vi "DC_Measurement.vi"(8 "stop":bool, 10 "millisecond multiple":u32, 11 "task/channels in":refnum<k21>="PTS_CAB1k_DCV") -> (0 "XY Graph":cluster{dbl[], dbl[]}(graph))   [LabVIEW 2021]
uses:
  <vilib>/DAQmx/read.llb/DAQmx Read (Analog 1D Wfm NChan NSamp).vi
  <vilib>/DAQmx/miscellaneous.llb/DAQmx Fill In Error Info.vi
  <vilib>/measure/madcrms.llb/Averaged DC-RMS for N Chan.vi
  <vilib>/measure/madcrms.llb/Basic Averaged DC-RMS for N Chan.vi
  <vilib>/measure/NI_MAPro.lvlib
panel:
  out "Waveform Graph":dbl[](graph)
  out "Array":dbl[](array[numeric])
  out "cycle average":dbl[](array[numeric]) format="%.2p"
  out "Raw Readings":waveform(dbl)[](graph)
  out "DC value waveforms":waveform(dbl)[](array[waveform])
  out "RMS value waveforms":waveform(dbl)[](array[waveform])
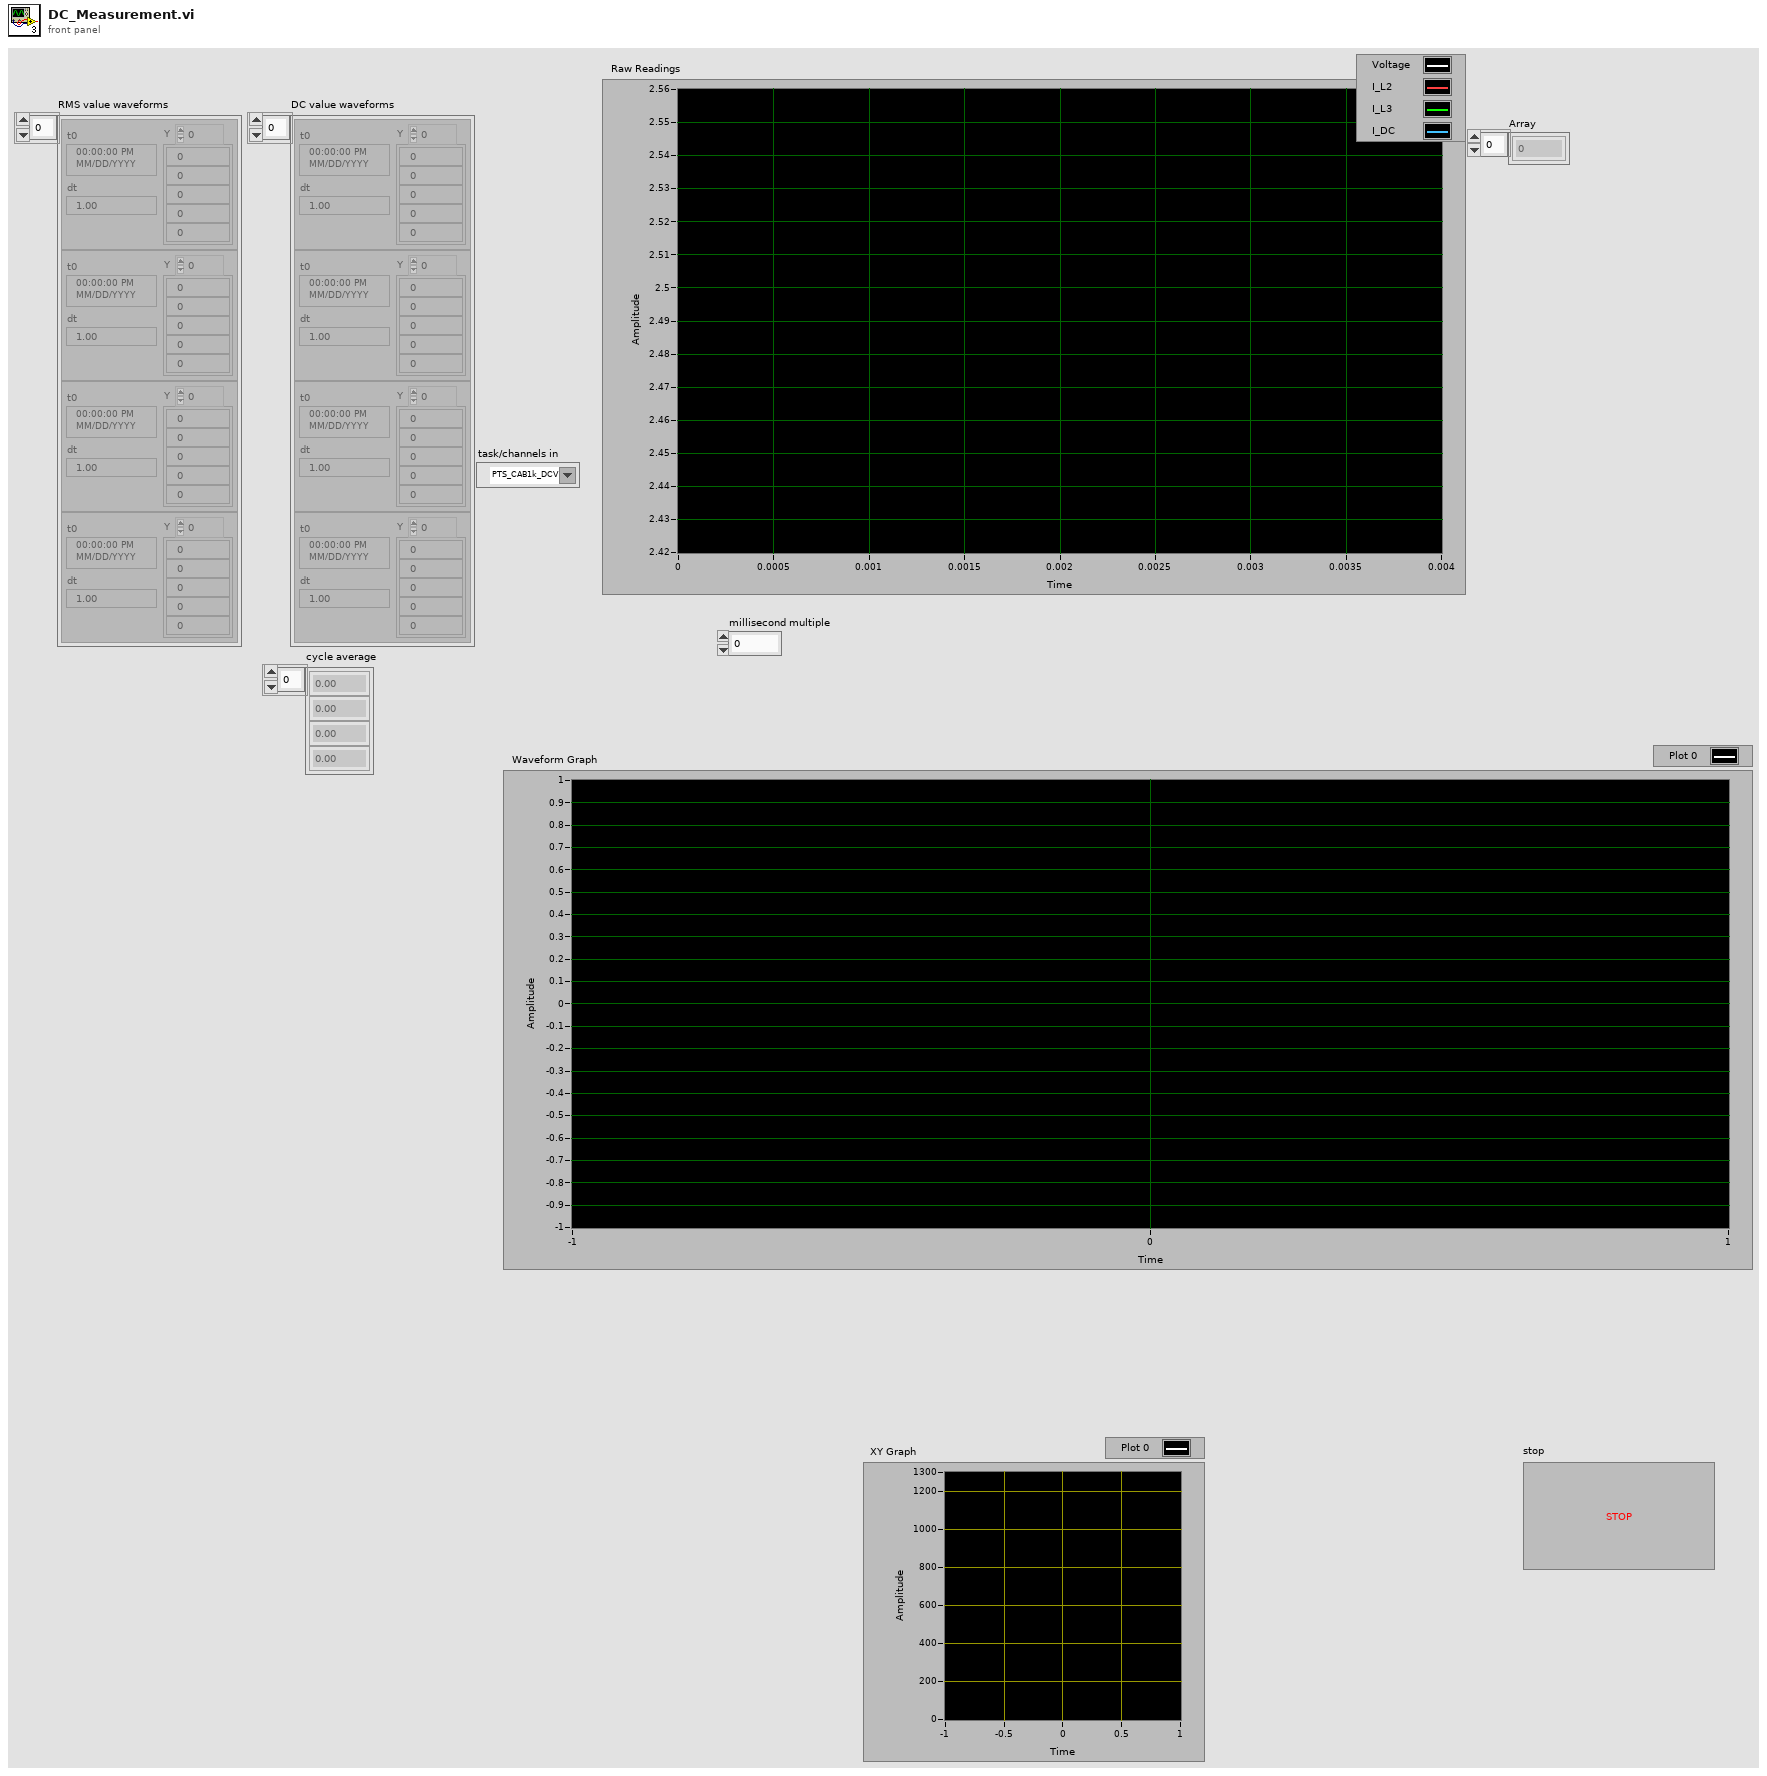
[diagram p1: front panel]
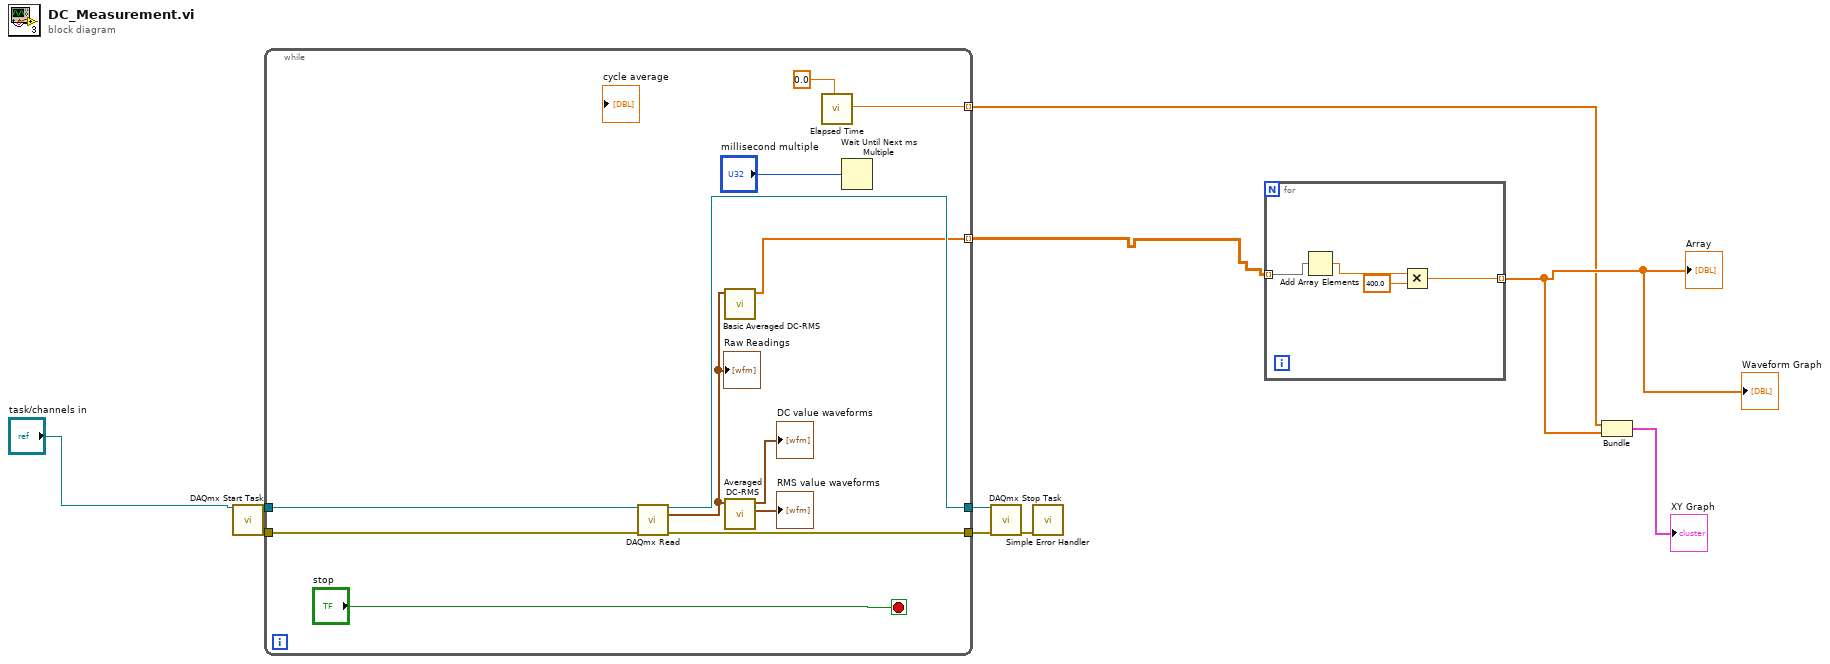
[diagram p0: block diagram]
diagram:
  n1 = call <vilib>:"DAQmx Start Task.vi"("task/channels in"="task/channels in") -> ("task out"=w10:refnum<k21>, "error out"=w8:errorcluster)  [unwired: 13 in]
  n2 = while {
    tunnel: w8 -> [w20]
    tunnel: [w19] -> w7
    tunnel: w10 -> [w22]
    tunnel: [w21] -> w9
    tunnel: [w14] -> w5 mode=indexing
    tunnel: [w12] -> w2 mode=indexing
    stop <- "stop" stop-if-true
    n3 = call-poly <vilib>:"DAQmx Read.vi"("task/channels in"=w22, "error in"=w20) -> ("task out"=w21:refnum<k21>, "data"=w15:waveform(dbl)[], "error out"=w19:errorcluster)  [unwired: 11 in]
    "Raw Readings" <- w15
    n4 = call-poly <vilib>:"Basic Averaged DC-RMS.vi"("signals in"=w15) -> ("DC values"=w14:dbl[])  [unwired: 7 in, 3 out]
    n5 = call-poly <vilib>:"Averaged DC-RMS.vi"("signals in"=w15) -> ("RMS value waveforms"=→"RMS value waveforms":waveform(dbl)[], "DC value waveforms"=→"DC value waveforms":waveform(dbl)[])  [unwired: 6 in, 3 out]
    n6 = call "Elapsed Time"("Set Start Time (s)"=0.0) -> ("Elapsed Time (s)"=w12:dbl)  [unwired: 11 in, 7 out]
    n7 = Wait Until Next ms Multiple(millisecond multiple="millisecond multiple") -> ()  [unwired: 1 out]
  }
  n8 = call <vilib>:"DAQmx Stop Task.vi"("task/channels in"=w9, "error in"=w7) -> ("error out"=w6:errorcluster)  [unwired: 12 in, 1 out]
  n9 = call <vilib>:"Simple Error Handler.vi"("error in (no error)"=w6) -> ()  [unwired: 4 in, 5 out]
  n10 = for {
    tunnel: w5 -> [w26] mode=indexing
    tunnel: [w23] -> w3 mode=indexing
    n11 = Add Array Elements(numeric array=w26) -> (sum=w25:dbl)
    n12 = Multiply(x=w25, y=400.0) -> (x*y=w23:dbl)
  }
  "Array" <- w3
  "Waveform Graph" <- w3
  n13 = Bundle(w2, w3) -> (→"XY Graph":cluster{dbl[], dbl[]})  [unwired: 1 in]
